vi "Configure Reference Waveform (Position).vi"(5 "Y Scale (1 V)":dbl=1.0, 6 "Y Range (1 V)":dbl=1.0, 7 "Y Offset (0 V)":dbl, 8 "error in (no error)":errorcluster, 9 "Skew (0 S)":dbl, 10 "Reference Waveform Location (1: Memory Location 1)":i32(ring)=1 items=["Memory Location 1"=1, "Memory Location 2"=2], 11 "VISA resource name":refnum<visa-resource-name>) -> (0 "error out":errorcluster, 3 "VISA resource name out":refnum<visa-resource-name>)   [LabVIEW 2015, in "Agilent 2000 3000 X-Series.lvlib"]
doc: "Configures position settings for reference waveform."
uses:
  <instrlib>/Agilent 2000 3000 X-Series/Agilent 2000 3000 X-Series.lvlib
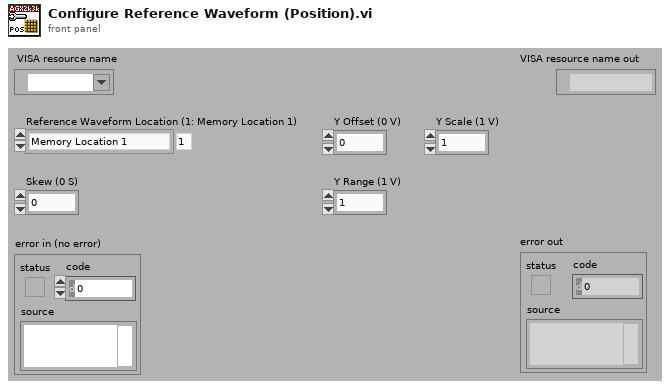
[diagram p1: front panel]
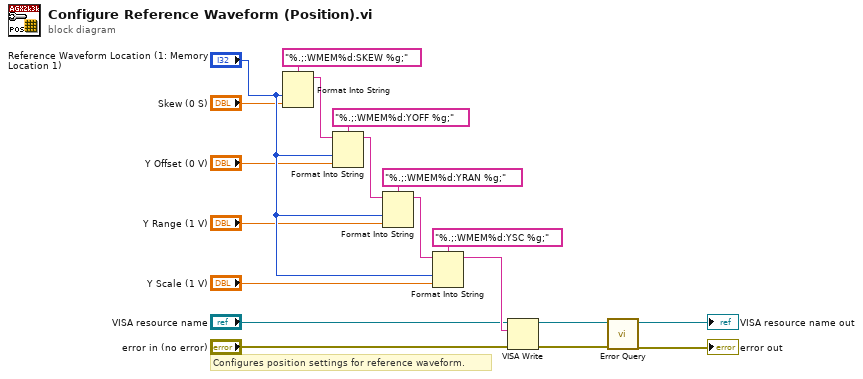
[diagram p0: block diagram]
diagram:
  # "Configures position settings for reference waveform."
  n1 = Format Into String(format string="%.;:WMEM%d:SKEW %g;", "Reference Waveform Location (1: Memory Location 1)", "Skew (0 S)") -> (resulting string=w16:string)  [unwired: 2 in, 1 out]
  n2 = Format Into String(format string="%.;:WMEM%d:YOFF %g;", initial string=w16, "Reference Waveform Location (1: Memory Location 1)", "Y Offset (0 V)") -> (resulting string=w13:string)  [unwired: 1 in, 1 out]
  n3 = Format Into String(format string="%.;:WMEM%d:YRAN %g;", initial string=w13, "Reference Waveform Location (1: Memory Location 1)", "Y Range (1 V)") -> (resulting string=w10:string)  [unwired: 1 in, 1 out]
  n4 = Format Into String(format string="%.;:WMEM%d:YSC %g;", initial string=w10, "Reference Waveform Location (1: Memory Location 1)", "Y Scale (1 V)") -> (resulting string=w7:string)  [unwired: 1 in, 1 out]
  n5 = VISA Write(VISA resource name="VISA resource name", write buffer=w7, error in (no error)="error in (no error)") -> (VISA resource name out=w4:refnum<visa-resource-name>, error out=w3:errorcluster)  [unwired: 1 out]
  n6 = call <instrlib>:"Error Query.vi"("error in (no error)"=w3, "VISA resource name"=w4) -> ("error out"=→"error out":errorcluster, "VISA resource name out"=→"VISA resource name out":refnum<visa-resource-name>)  [unwired: 8 out]
